vi "3.9.3-Zero Crossing.vi"(1 "Signal Out":dbl) -> (0 "Boolean":bool)   [LabVIEW 2010]
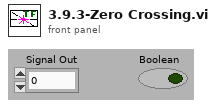
[diagram p1: front panel]
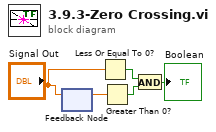
[diagram p0: block diagram]
diagram:
  n1 = feedback #1() -> (w1:dbl)  [unwired: 1 in]
  n2 = feedback-in #1("Signal Out") -> ()
  n3 = Less Or Equal To 0?(x="Signal Out") -> (x <= 0?=w4:bool)
  n4 = Greater Than 0?(x=w1) -> (x > 0?=w3:bool)
  n5 = And(x=w4, y=w3) -> (x .and. y?=→"Boolean":bool)
